vi "Named_Serial_Comms.vi"(0 "Channel Name":string, 1 "Write":string, 2 "Timeout/ms":u32=500, 4 "!Error retries":i32=10, 6 "!Timeout retries":i32=3, 9 "Port Name":string, 11 "Term Grep":string="\r$", 12 "Log Errors?":bool=TRUE, 13 "Terminate Count":i32) -> (3 "Read":string="This is simulation mode", 10 "millisecond timer value":u32, 14 "Timed out":bool, 15 "Serial Error":bool)   [LabVIEW 2016]
doc: "The Serial Communication VI performs bidirectional communication with a port. It initializes the port, writes a string to the port, and performs a read with timeout. The Read with Timeout will wait until a terminating character is received or the time limit is up, whichever comes first.\nThe initialisation parameters, terminating character, and timeout, are all set in the Serial Setup Global."
uses:
  Port_Params.ctl
  <vilib>/Instr/_visa.llb/VISA Find Search Mode.ctl
  <vilib>/Instr/serial.llb/serpConfig.vi
panel:
  in  "Tab Control":T1(tab)
  in  "Uppercase?":bool
  in  "Append Return?":bool
  in  "!stop":bool
  out "Terminated?":bool
  in  "Force setup reload":bool
  in  "Save Setups?":bool
  out "Buffer Trash":string
  out "byte count":u32
  out "Error Description":string
  out "Port Settings Array":T2[](array[typedef]) {"flow control etc."."parity err byte" format="%.0x"; "flow control etc."."XON byte" format="%.0x"; "flow control etc."."XOFF byte" format="%.0x"; "data bits" min=5 max=8 step=1}
  out "enumerated ports":string[](array[string])
  out "Ports having file settings":string[](array[string])
  out "Port Initialised?":bool[](array[boolean])
  out "Setting Number":i32
  out "Port Initialisation Parameters":T2={"Name"="", "flow control etc."={"input XON/XOFF"=FALSE, "input HW Handshake"=FALSE, "input alt HW HShk"=FALSE, "output XON/XOFF"=FALSE, "output HW Handshake"=FALSE, "output alt HW HShk"=FALSE, "XOFF byte "=0, "XON byte"=0, "parity err byte"=0}, "buffer size"=0, "baud rate"=9600, "data bits"=8, "stop bits"=enum."1 bit", "parity"=enum."no parity"} {"flow control etc."."parity err byte" format="%.0x"; "flow control etc."."XON byte" format="%.0x"; "flow control etc."."XOFF byte" format="%.0x"; "data bits" min=5 max=8 step=1}
  out "isGillUsonic":bool
  out "etherComms":errorcluster
  out "Audit trail":string[](array[string])
  out "Case":string="Simulate"
  out "Initialise error":i32
  out "Write error":i32
  out "n-bytes error code":i32
  out "read error code":i32
  out "Close Port error":i32
  out "load setups error":bool
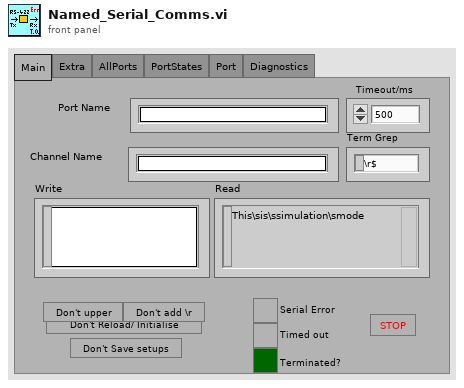
[diagram p1: front panel]
types:
  T1 = enum32{"Main", "Extra", "AllPorts", "PortStates", "Port", "Diagnostics"}
  T2 = typedef "Port_Params.ctl" = cluster{"Name":string, "flow control etc.":cluster{"input XON/XOFF":bool, "input HW Handshake":bool, "input alt HW HShk":bool, "output XON/XOFF":bool, "output HW Handshake":bool, "output alt HW HShk":bool, "XOFF byte ":u8, "XON byte":u8, "parity err byte":u16}, "buffer size":u16, "baud rate":u32, "data bits":u16, "stop bits":enum16{"1 bit", "1.5 bits", "2 bits"}, "parity":enum16{"no parity", "odd parity", "even parity", "mark parity", "space parity"}}
  T3 = enum16{"Standard", "Buffered", "CRLF", "Immediate"}
  T4 = typedef "VISA Find Search Mode.ctl" = u32
  T5 = cluster{"input XON/XOFF":bool, "input HW Handshake":bool, "input alt HW HShk":bool, "output XON/XOFF":bool, "output HW Handshake":bool, "output alt HW HShk":bool, "XOFF byte ":u8, "XON byte":u8, "parity err byte":u16}
  T6 = enum16{"no parity", "odd parity", "even parity", "mark parity", "space parity"}
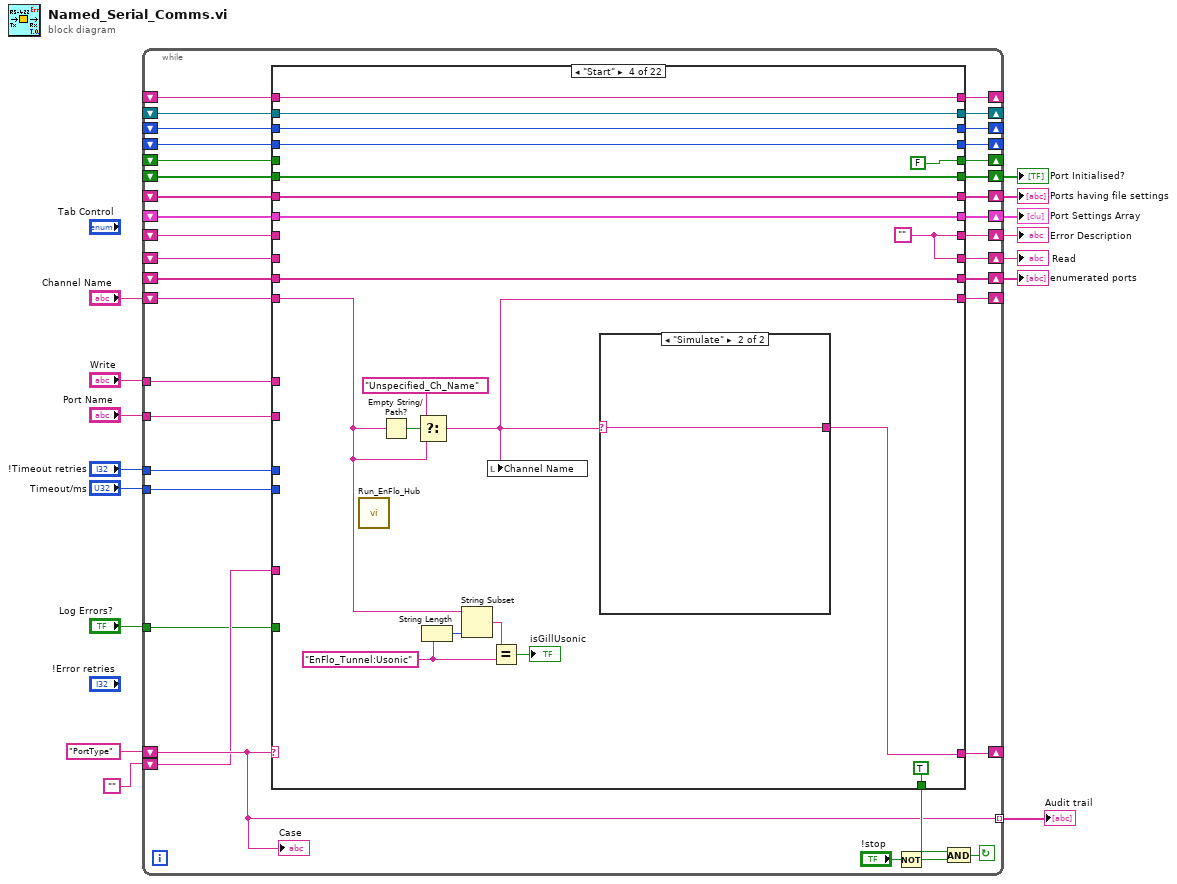
[diagram p0: block diagram]
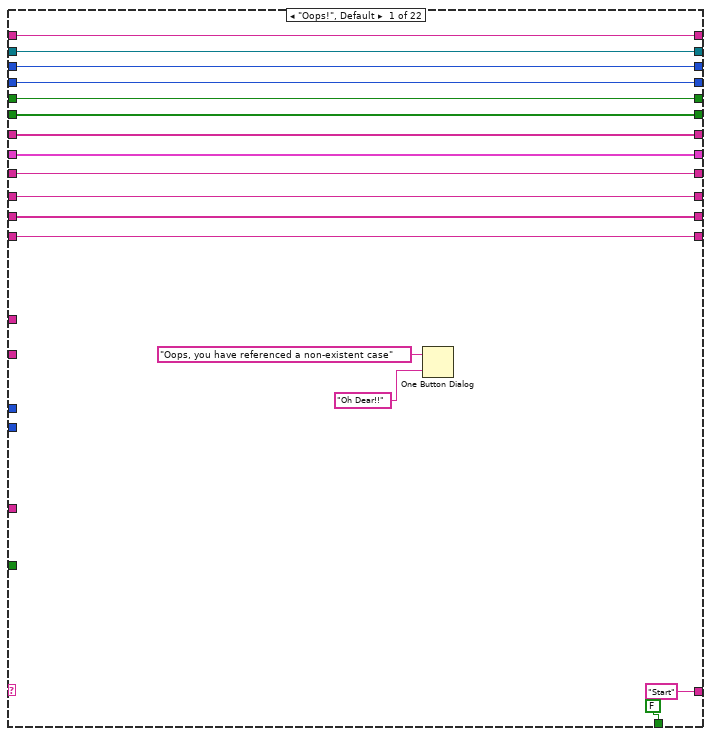
[diagram p2: hidden frame]
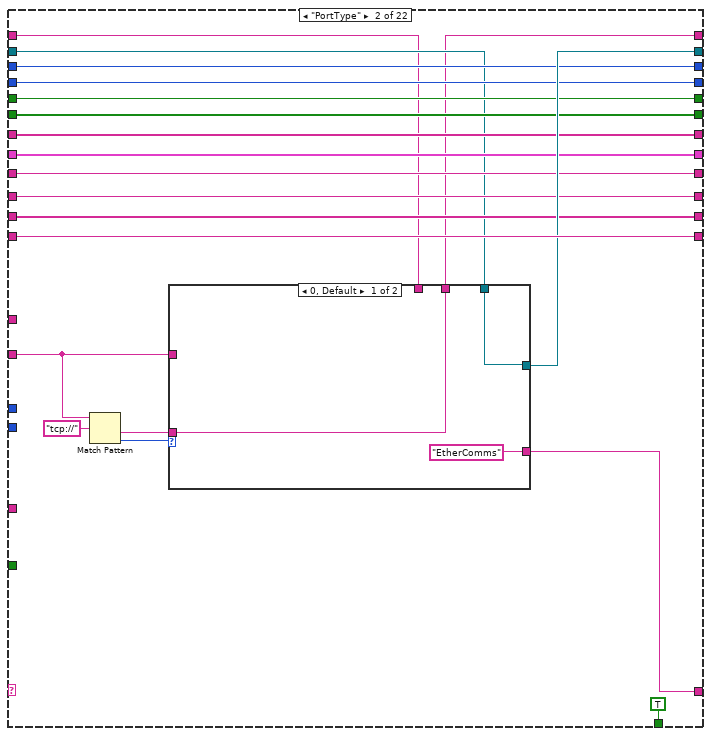
[diagram p3: hidden frame]
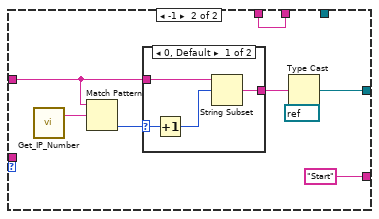
[diagram p4: hidden frame]
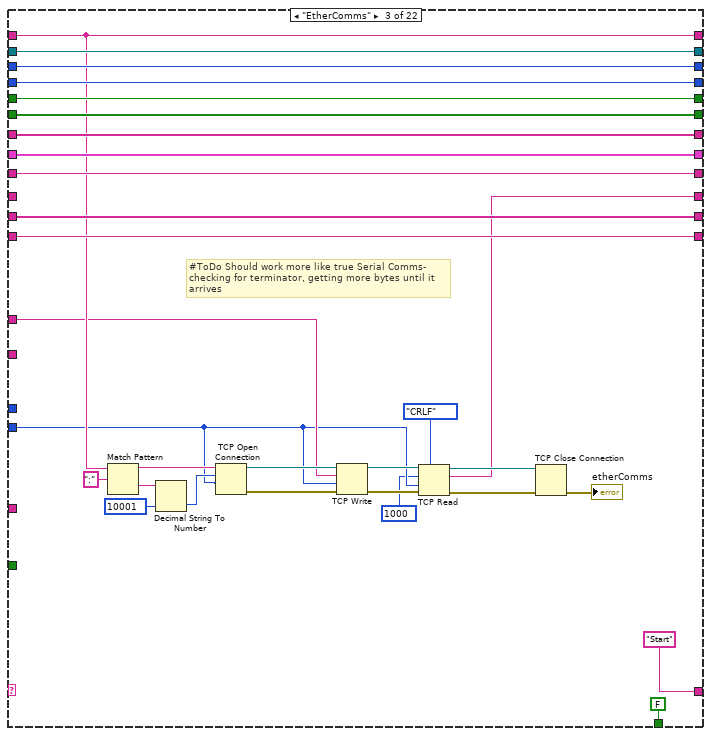
[diagram p6: hidden frame]
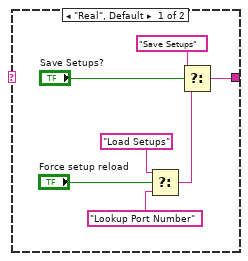
[diagram p7: hidden frame]
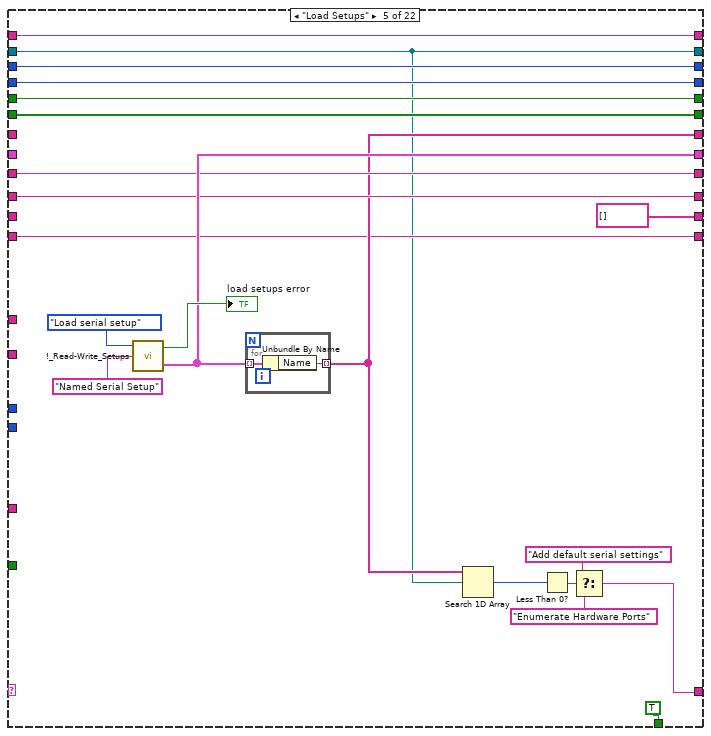
[diagram p8: hidden frame]
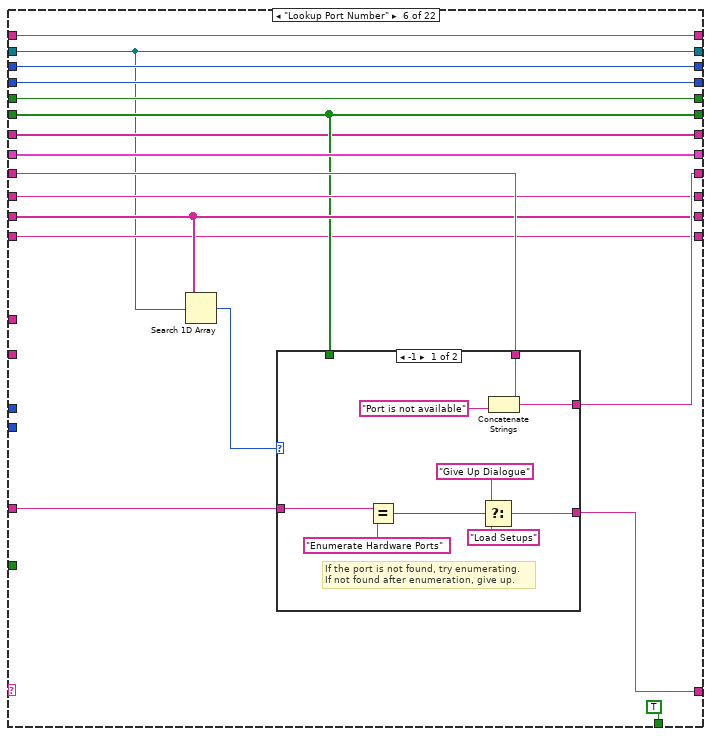
[diagram p9: hidden frame]
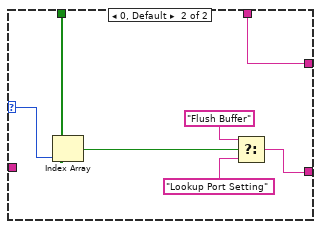
[diagram p10: hidden frame]
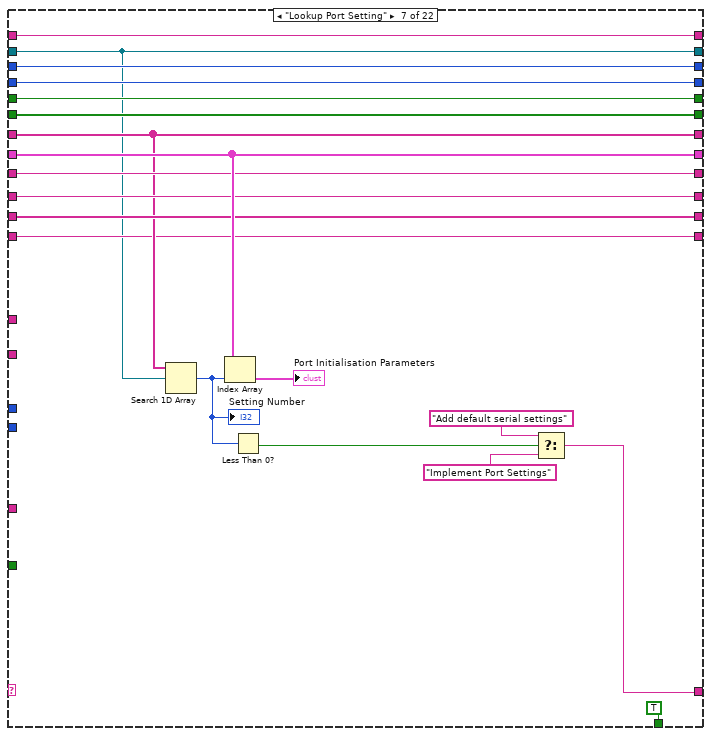
[diagram p11: hidden frame]
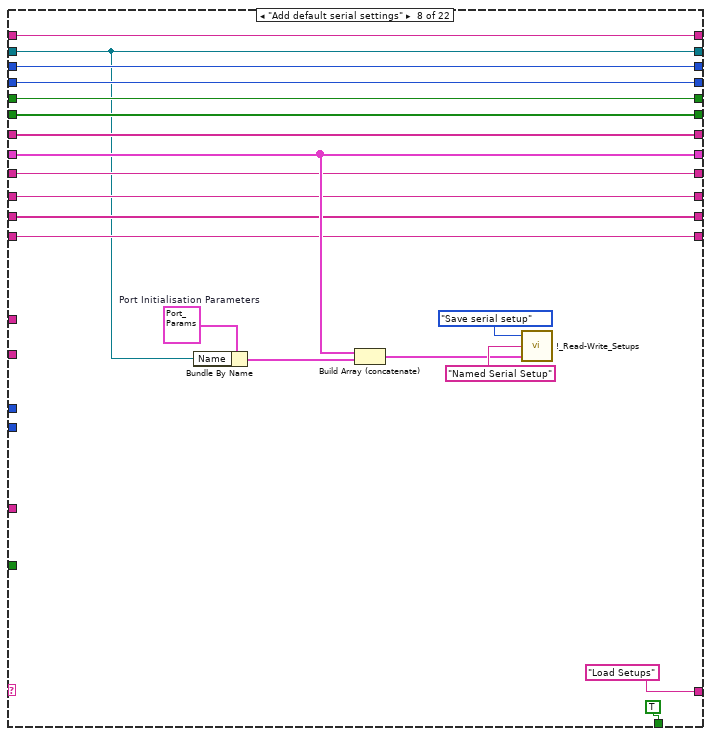
[diagram p12: hidden frame]
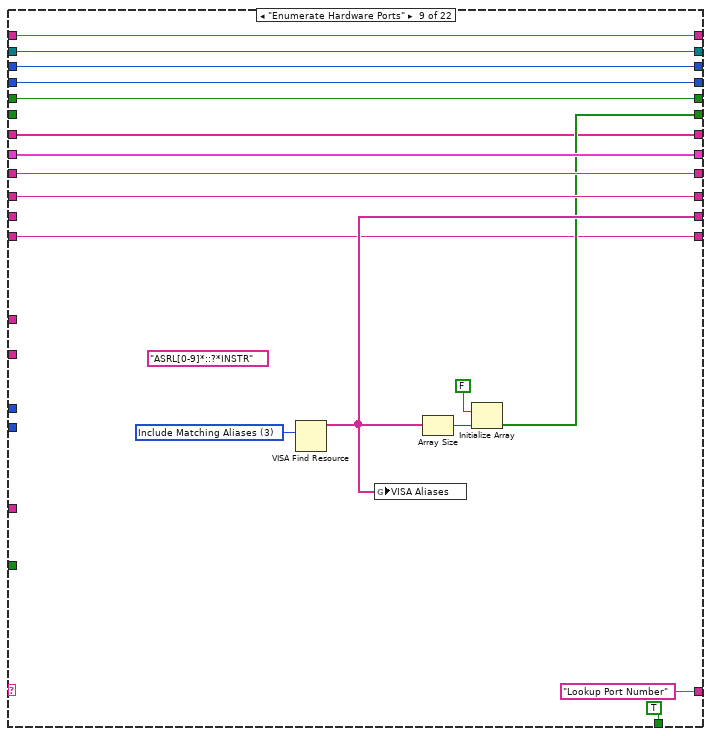
[diagram p13: hidden frame]
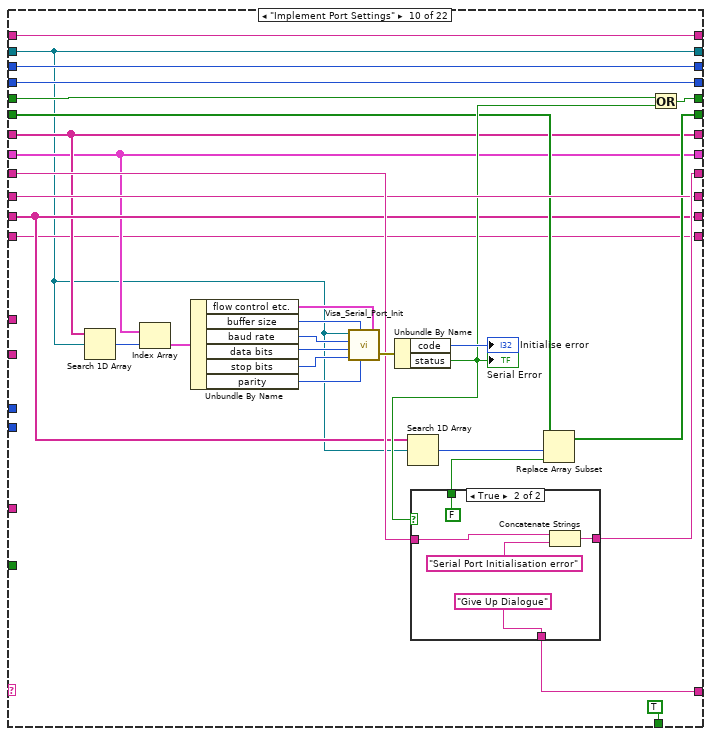
[diagram p14: hidden frame]
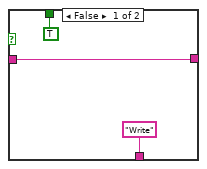
[diagram p15: hidden frame]
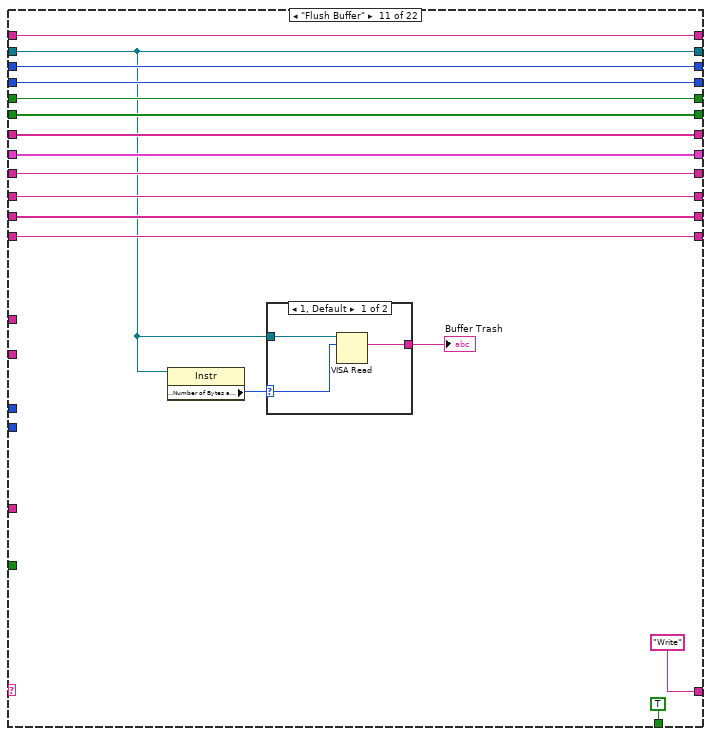
[diagram p16: hidden frame]
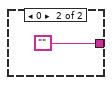
[diagram p17: hidden frame]
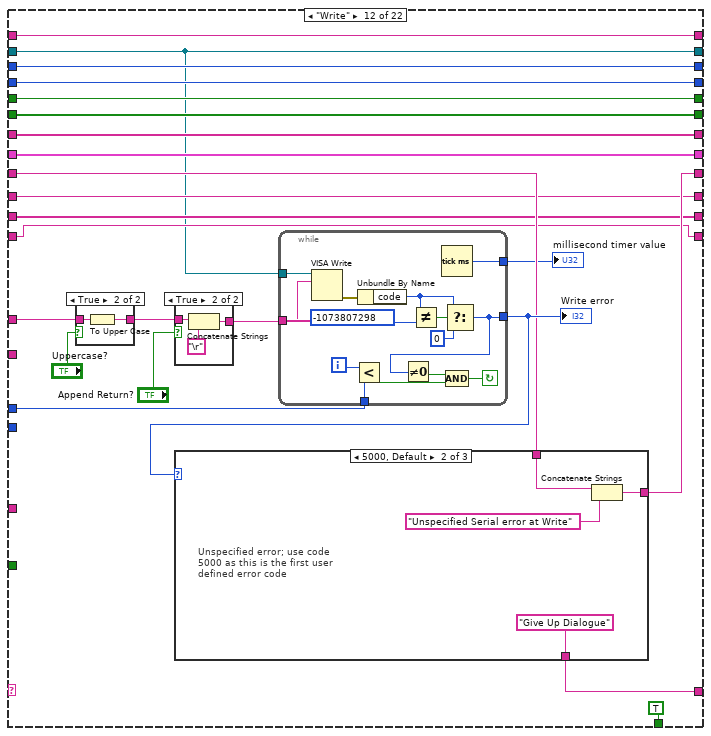
[diagram p18: hidden frame]
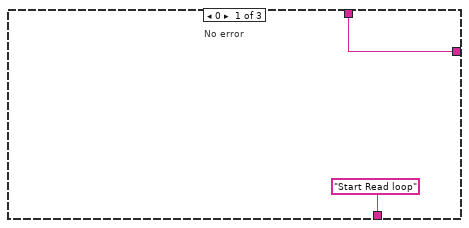
[diagram p19: hidden frame]
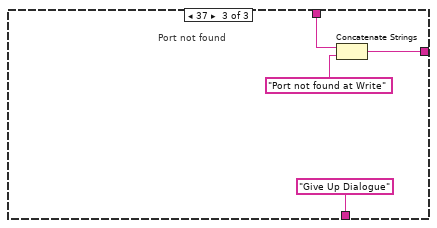
[diagram p20: hidden frame]
diagram:
  n1 = while {
    tunnel: "!Timeout retries" -> [w43]
    shift-left: "" -> [w44]
    tunnel: [w45] -> w3 mode=indexing
    shift-left: "PortType" -> [w45]
    shift-right: [w46] -> _
    tunnel: "Write" -> [w51]
    tunnel: "Log Errors?" -> [w42]
    shift-right: [w41] -> w10
    shift-left: _ -> [w40]
    shift-right: [w38] -> w9
    shift-left: _ -> [w39]
    shift-right: [w37] -> w8
    shift-left: _ -> [w36]
    shift-right: [w35] -> w7
    shift-left: _ -> [w34]
    shift-right: [w33] -> _
    shift-left: _ -> [w32]
    shift-right: [w31] -> w6
    shift-left: _ -> [w30]
    shift-right: [w28] -> w5
    shift-left: _ -> [w29]
    shift-right: [w25] -> _
    shift-left: _ -> [w24]
    shift-right: [w27] -> _
    shift-left: _ -> [w26]
    shift-right: [w22] -> _
    shift-left: "Channel Name" -> [w23]
    shift-right: [w21] -> _
    shift-left: _ -> [w20]
    tunnel: "Port Name" -> [w19]
    shift-right: [w18] -> _
    shift-left: _ -> [w17]
    tunnel: "Timeout/ms" -> [w16]
    stop <- w49 continue-if-true
    n2 = case shown="\"Start\"" w45 {
      tunnel: w51 -> [_ _ w109 _ _ _ _ _ _ _ _ w350 _ _ _ _ _ w532 w558 _ _ _]
      tunnel: ["Start" ("f") w68 "Start" w153 w164 w200 w220 "Load Setups" ("f") "Lookup Port Number" w295 "Write" ("f") w347 "Bytes At Serial Port?" ("f") w412 w454 w480 w522 "Start" "Start" "Start" "Start" ("f") "Load Setups" ("f")] -> w46
      tunnel: [FALSE TRUE FALSE TRUE TRUE TRUE TRUE TRUE TRUE TRUE TRUE TRUE TRUE TRUE TRUE TRUE TRUE FALSE FALSE TRUE FALSE TRUE] -> w50
      tunnel: w44 -> [_ _ _ _ _ w199 _ _ _ _ _ _ _ _ _ _ _ _ _ _ _ _]
      tunnel: w43 -> [_ _ _ _ _ _ _ _ _ _ _ w345 _ w411 _ _ _ _ _ _ _ _]
      tunnel: w42 -> [_ _ _ _ _ _ _ _ _ _ _ _ _ _ _ _ _ w538 _ _ _ _]
      tunnel: [w63 w80 w127 w151 w178 w198 w233 w248 w268 w279 w324 w344 w396 w410 w446 w473 w518 w537 w555 w574 w591 w605] -> w41
      tunnel: w40 -> [w63 w80 w127 w151 _ w198 w233 w248 w268 w279 w324 w344 w396 w410 w446 w473 w518 w537 w555 w574 w591 w605]
      tunnel: w39 -> [w62 w79 w126 _ w177 w197 w232 w247 w267 w290 w323 w342 w395 w409 w445 w472 w517 w536 w554 w573 w590 w604]
      tunnel: [w62 w79 w126 w150 w177 w196 w232 w247 w267 w291 w323 w343 w395 w409 w445 w472 w517 w536 w554 w573 w590 w604] -> w38
      tunnel: [w61 w78 w105 w150 w176 w195 w231 w246 w266 w289 w322 w341 "" w408 w444 w471 w516 w535 w553 w572 "Simulated Serial Read" w603] -> w37
      tunnel: w36 -> [w61 w78 _ _ w176 w195 w231 w246 w266 w289 w322 w341 _ w408 w443 w471 w516 w535 w553 w572 _ w603]
      tunnel: [w60 w77 w125 w149 string[] [] ("enumerated ports") w194 w230 w245 w265 w281 w321 w340 w393 w407 w442 w470 w515 w534 w552 w571 w588 w602] -> w35
      tunnel: w34 -> [w60 w77 w125 w149 _ w194 w230 w245 _ w281 w321 w340 w393 w407 w442 w470 w515 w534 w552 w571 w588 w602]
      tunnel: [w59 w83 w130 FALSE w174 w193 w229 w244 w264 w287 w318 w339 w392 w406 w441 w469 w513 w533 w551 w570 w587 w601] -> w33
      tunnel: w32 -> [w59 w83 w130 _ w174 w193 w229 w244 w264 w288 w318 w339 w392 w406 w441 w469 w514 w533 w551 w570 w587 w601]
      tunnel: [w58 w82 w129 w147 w173 w191 w228 w243 w263 w284 w317 w338 w391 w405 w440 w468 w511 w531 w550 w569 w586 w600] -> w31
      tunnel: w30 -> [w58 w82 w129 w147 w173 w191 w228 w243 _ w283 w317 w338 w391 w405 w440 w468 w511 w531 w550 w569 w586 w600]
      tunnel: [w57 w81 w128 w146 w172 w190 w227 w242 w262 w280 w316 w337 w390 w404 w439 w467 w510 w530 w549 w568 w585 w599] -> w28
      tunnel: w29 -> [w57 w81 w128 w146 _ w190 w227 w242 w262 w280 w316 w337 w390 w404 w439 w467 w510 w530 w549 w568 w585 w599]
      tunnel: [w56 w85 w132 w145 w171 w189 w226 w241 w261 w277 w315 w336 w389 w402 w435 w466 w509 w529 w548 w567 w584 w598] -> w27
      tunnel: w26 -> [w56 w85 w132 w145 w171 w189 w226 w241 w261 w277 w315 w336 _ w402 w435 w466 w509 w529 w548 w567 w584 w598]
      tunnel: [w55 w84 w131 w144 w170 w188 w225 w240 w260 w276 w314 w335 w388 w403 w434 w465 w508 w528 w547 w566 w583 w597] -> w25
      tunnel: w24 -> [w55 w84 w131 w144 w170 w188 w225 w240 w260 w276 w314 w335 w388 _ w434 w465 w508 w528 w547 w566 w583 w597]
      tunnel: w23 -> [w54 w87 w133 w136 w169 w187 w224 w239 w258 w275 w313 w333 w387 w401 w433 w464 w507 w527 w543 w565 w582 w596]
      tunnel: [w54 w87 w133 w134 w169 w187 w224 w239 w258 w275 w313 w333 w387 w401 w433 w464 w507 w527 w543 w565 w582 w596] -> w22
      tunnel: [w53 w86 w122 w141 w163 w186 w219 w238 w257 w274 w312 w332 w386 w400 w432 w463 w506 w526 w542 w564 w581 w595] -> w21
      tunnel: w20 -> [w53 w71 w122 w141 w163 w186 w219 w238 w257 w274 w312 w332 w386 w400 w432 w463 w506 w526 w542 w564 w581 w595]
      tunnel: w19 -> [_ w75 _ _ _ _ _ _ _ _ _ _ _ _ _ _ _ _ _ _ _ _]
      tunnel: [w52 w70 w115 w140 w162 w185 w218 w237 w256 w273 w311 w331 w385 w399 w431 w462 w505 w525 w541 w563 w580 w594] -> w18
      tunnel: w17 -> [w52 w69 w115 w140 w162 w185 w218 w237 w256 w273 w311 w331 w385 w399 w431 w462 w505 w525 w541 w563 w580 w594]
      tunnel: w16 -> [_ _ w108 _ _ _ _ _ _ _ _ _ _ _ _ _ w504 _ _ _ _ _]
      frame "Oops!", Default {
        n3 = One Button Dialog(message="Oops, you have referenced a non-existent case", button name ("OK")="Oh Dear!!") -> ()  [unwired: 1 out]
      }
      frame "PortType" {
        n4 = Match Pattern(string=w75, regular expression="tcp://") -> (after substring=w72:string, offset past match=w73:i32)  [unwired: 1 in, 2 out]
        n5 = case shown="0, Default" w73 {
          tunnel: [w90 w94] -> w86
          tunnel: w75 -> [_ w93]
          tunnel: w72 -> [w89 _]
          tunnel: w71 -> [w90 _]
          tunnel: [w89 w92] -> w70
          tunnel: w69 -> [_ w92]
          tunnel: ["EtherComms" "Start"] -> w68
          frame 0, Default {
          }
          frame -1 {
            n6 = call "Get_IP_Number.vi"() -> ("IP Number"=w97:string)  [unwired: 1 out]
            n7 = Match Pattern(string=w93, regular expression=w97) -> (offset past match=w96:i32)  [unwired: 4 out]
            n8 = case shown="0, Default" w96 {
              selector: w96 -> [w99 _]
              tunnel: [w100 w103] -> w98
              tunnel: w93 -> [w101 w103]
              frame 0, Default {
                n9 = Increment(x=w99) -> (x+1=w102:i32)
                n10 = String Subset(string=w101, offset (0)=w102) -> (substring=w100:string)  [unwired: 1 out]
              }
              frame -1 {
              }
            }
            n11 = Type Cast(type=refnum<visa-resource-name> refnum ("dup VISA resource name"), x=w98) -> (*(type *) &x=w94:refnum<visa-resource-name>)
          }
        }
      }
      frame "EtherComms" {
        # "#ToDo Should work more like true Serial Comms- checking for terminator, getting more bytes until it arrives"
        n12 = Match Pattern(string=w115, regular expression=":") -> (before substring=w113:string, after substring=w112:string)  [unwired: 1 in, 2 out]
        n13 = Decimal String To Number(string=w112, default (0L)=u16 10001 ("default (0 I32)")) -> (number=w111:u16)  [unwired: 1 in, 1 out]
        n14 = TCP Open Connection(address=w113, remote port or service name=w111, timeout ms (60000)=w108) -> (connection ID=w116:refnum<k5>, error out=w119:errorcluster)  [unwired: 2 in]
        n15 = TCP Write(connection ID=w116, data in=w109, error in (no error)=w119, 9:w108) -> (connection ID out=w117:refnum<k5>, error out=w118:errorcluster)  [unwired: 1 out]
        n16 = TCP Read(connection ID=w117, bytes to read=1000, error in (no error)=w118, 7:T3."CRLF" ("mode (standard)"), 9:w108) -> (connection ID out=w121:refnum<k5>, data out=w105:string, error out=w120:errorcluster)
        n17 = TCP Close Connection(connection ID=w121, error in (no error)=w120) -> (error out=→"etherComms":errorcluster)  [unwired: 1 in, 1 out]
      }
      frame "Start" {
        w139 = "EnFlo_Tunnel:Usonic"
        w150 = ""
        n18 = call "Run_EnFlo_Hub.vi"() -> ()  [unwired: 1 in, 7 out]
        n19 = Empty String/Path?(string/path=w136) -> (empty?=w143:bool)
        n20 = Select(t="Unspecified_Ch_Name", s=w143, f=w136) -> (s? t:f=w134:string)
        n21 = String Length(string=w139) -> (length=w137:i32)
        n22 = String Subset(string=w136, length (rest)=w137) -> (substring=w138:string)  [unwired: 1 out]
        n23 = local write "Channel Name"(w134) -> ()
        n24 = Equal?(x=w138, y=w139) -> (x = y?=→"isGillUsonic":bool)
        n25 = case shown="\"Simulate\"" w134 {
          selector: w134 -> [_ w161]
          tunnel: [w156 w161] -> w153
          frame "Real", Default {
            n26 = Select(t="Load Setups" ("f"), s="Force setup reload", f="Lookup Port Number") -> (s? t:f=w157:string)
            n27 = Select(t="Save Setups", s="Save Setups?", f=w157) -> (s? t:f=w156:string)
          }
          frame "Simulate" {
          }
        }
      }
      frame "Load Setups" {
        n28 = call "!_Read-Write_Setups.vi"("Setup Name"="Named Serial Setup", "Mode"=enum16{"Load serial setup", "Save serial setup"}."Load serial setup") -> ("Port Settings Array Out"=w178:T2[], "error unflattening"=→"load setups error":bool)  [unwired: 1 in]
        n29 = for {
          tunnel: w178 -> [w184] mode=indexing
          tunnel: [w183] -> w172 mode=indexing
          n30 = Unbundle By Name(w184) -> ("Name"=w183:string)
        }
        n31 = Search 1D Array(1D array=w172, element=w163) -> (index of element=w168:i32)  [unwired: 1 out]
        n32 = Less Than 0?(x=w168) -> (x < 0?=w167:bool)
        n33 = Select(t="Add default serial settings", s=w167, f="Enumerate Hardware Ports") -> (s? t:f=w164:string)
      }
      frame "Lookup Port Number" {
        n34 = Search 1D Array(1D array=w194, element=w186) -> (index of element=w192:i32)  [unwired: 1 out]
        n35 = case shown="-1" w192 {
          selector: w192 -> [_ w211]
          tunnel: [w210 w217] -> w200
          tunnel: w199 -> [w207 _]
          tunnel: w197 -> [w203 w213]
          tunnel: [w202 w213] -> w196
          tunnel: w191 -> [_ w212]
          frame -1 {
            # "If the port is not found, try enumerating.\nIf not found after enumeration, give up."
            n36 = Equal?(x=w207, y="Enumerate Hardware Ports" ("f")) -> (x = y?=w209:bool)
            n37 = Select(t="Give Up Dialogue" ("f"), s=w209, f="Load Setups") -> (s? t:f=w210:string)
            n38 = Concatenate Strings(w203, "Port is not available" ("Error Description")) -> (w202:string)
          }
          frame 0, Default {
            n39 = Index Array(array=w212, index=w211) -> (element=w216:bool)
            n40 = Select(t="Flush Buffer" ("f"), s=w216, f="Lookup Port Setting") -> (s? t:f=w217:string)
          }
        }
      }
      frame "Lookup Port Setting" {
        n41 = Search 1D Array(1D array=w227, element=w219) -> (index of element=w234:i32)  [unwired: 1 out]
        "Setting Number" <- w234
        n42 = Index Array(array=w233, index=w234) -> (element=→"Port Initialisation Parameters":T2)
        n43 = Less Than 0?(x=w234) -> (x < 0?=w223:bool)
        n44 = Select(t="Add default serial settings", s=w223, f="Implement Port Settings") -> (s? t:f=w220:string)
      }
      frame "Add default serial settings" {
        w255 = T2 {"Name"="", "flow control etc."={"input XON/XOFF"=FALSE, "input HW Handshake"=FALSE, "input alt HW HShk"=FALSE, "output XON/XOFF"=FALSE, "output HW Handshake"=FALSE, "output alt HW HShk"=FALSE, "XOFF byte "=19, "XON byte"=17, "parity err byte"=0}, "buffer size"=200, "baud rate"=9600, "data bits"=8, "stop bits"=enum."1 bit", "parity"=enum."no parity"}  # Port Initialisation Parameters
        n45 = Bundle By Name(cluster=w255, "Name"=w238) -> (w254:T2)
        n46 = Build Array (concatenate)(w248, w254) -> (w251:T2[])
        n47 = call "!_Read-Write_Setups.vi"("Port Settings Array In"=w251, "Setup Name"="Named Serial Setup", "Mode"=enum16{"Load serial setup", "Save serial setup"}."Save serial setup") -> ()  [unwired: 2 out]
      }
      frame "Enumerate Hardware Ports" {
        w259 = T4 3 items=["Canonical Names Only"=0, "Aliases Only"=2, "Include Matching Aliases"=3, "Include All Aliases"=4] ("Search Mode")
        (unwired) "ASRL[0-9]*::?*INSTR" ("expression (\"?*\")")
        n48 = VISA Find Resource(10:w259) -> (3:w265:string[])  [unwired: 1 in, 3 out]
        n49 = global write "serpConfig.vi" "VISA Aliases"(w265) -> ()
        n50 = Array Size(array=w265) -> (size(s)=w270:i32)
        n51 = Initialize Array(FALSE, w270) -> (w263:bool[])
      }
      frame "Implement Port Settings" {
        n52 = Search 1D Array(1D array=w280, element=w274) -> (index of element=w282:i32)  [unwired: 1 out]
        n53 = Index Array(array=w279, index=w282) -> (element=w278:T2)
        n54 = Unbundle By Name(w278) -> ("flow control etc."=w302:T5, "buffer size"=w301:u16, "baud rate"=w300:u32, "data bits"=w299:u16, "stop bits"=w298:enum16{"1 bit", "1.5 bits", "2 bits"}, "parity"=w297:T6)
        n55 = call "Visa_Serial_Port_Init.vi"("flow control etc."=w302, "parity"=w297, "buffer size"=w301, "stop bits"=w298, "data bits"=w299, "baud rate"=w300, "Visa Port Name"=w274) -> ("error out"=w293:errorcluster)
        n56 = Unbundle By Name(w293) -> ("code"=→"Initialise error":i32, "status"=w286:bool)
        "Serial Error" <- w286
        n57 = Search 1D Array(1D array=w281, element=w274) -> (index of element=w285:i32)  [unwired: 1 out]
        n58 = case shown="True" w286 {
          tunnel: ["Write" "Give Up Dialogue"] -> w295
          tunnel: [TRUE ("Element Data") FALSE ("Element Data")] -> w294
          tunnel: [w303 w307] -> w291
          tunnel: w290 -> [w303 w306]
          frame False {
          }
          frame True {
            n59 = Concatenate Strings(w306, "Serial Port Initialisation error" ("Error Description")) -> (w307:string)
          }
        }
        n60 = Replace Array Subset(array=w283, new element=w294, index=w285) -> (w284:bool[])
        n61 = Or(x=w288, y=w286) -> (x .or. y?=w287:bool)
      }
      frame "Flush Buffer" {
        n62 = property class="Instr"(reference=w312) -> ("Serial Settings:Number of Bytes at Serial Port"=w320:u32)  [unwired: 1 in, 2 out]
        n63 = case shown="1, Default" w320 {
          selector: w320 -> [w327 _]
          tunnel: [w329 ""] -> w319
          tunnel: w312 -> [w328 _]
          frame 1, Default {
            n64 = VISA Read(VISA resource name=w328, byte count=w327) -> (read buffer=w329:string)  [unwired: 1 in, 3 out]
          }
          frame 0 {
          }
        }
        "Buffer Trash" <- w319
      }
      frame "Write" {
        n65 = case shown="True" "Uppercase?" {
          tunnel: w350 -> [w382 w384]
          tunnel: [w382 w383] -> w352
          frame False {
          }
          frame True {
            n66 = To Upper Case(1:w384) -> (0:w383:string)
          }
        }
        n67 = case shown="True" "Append Return?" {
          tunnel: w352 -> [w378 w381]
          tunnel: [w378 w380] -> w349
          frame False {
          }
          frame True {
            n68 = Concatenate Strings(w381, "\r") -> (w380:string)
          }
        }
        n69 = while {
          tunnel: w345 -> [w363]
          tunnel: [w354] -> w346
          tunnel: w349 -> [w361]
          tunnel: w332 -> [w360]
          tunnel: [w359] -> w334
          i -> [w367]
          stop <- w364 continue-if-true
          n70 = VISA Write(VISA resource name=w360, write buffer=w361) -> (error out=w362:errorcluster)  [unwired: 1 in, 2 out]
          n71 = Less?(x=w367, y=w363) -> (x < y?=w366:bool)
          n72 = Unbundle By Name(w362) -> ("code"=w356:i32)
          n73 = Not Equal?(x=w356, y=-1073807298 ("code")) -> (x != y?=w357:bool)
          n74 = Tick Count (ms)() -> (millisecond timer value=w359:u32)
          n75 = Select(t=w356, s=w357, f=0) -> (s? t:f=w354:i32)
          n76 = Not Equal To 0?(x=w354) -> (x != 0?=w365:bool)
          n77 = Compound Arithmetic op=AND(w365, w366) -> (w364:bool)
        }
        "Write error" <- w346
        "millisecond timer value" <- w334
        n78 = case shown="5000, Default" w346 {
          tunnel: ["Start Read loop" "Give Up Dialogue" "Give Up Dialogue"] -> w347
          tunnel: [w368 w371 w374] -> w343
          tunnel: w342 -> [w368 w370 w376]
          frame 0 {
            # "No error"
          }
          frame 5000, Default {
            # "Unspecified error; use code 5000 as this is the first user defined error code"
            n79 = Concatenate Strings(w370, "Unspecified Serial error at Write" ("Error Description")) -> (w371:string)
          }
          frame 37 {
            # "Port not found"
            n80 = Concatenate Strings(w376, "Port not found at Write" ("Error Description")) -> (w374:string)
          }
        }
      }
      frame "Start Read loop" {
        n81 = Tick Count (ms)() -> (millisecond timer value=w389:u32)
      }
      frame "Bytes At Serial Port?" {
        # "#Yuk Shouldn't use \"Timeout retries\" to say how many times to check for bytes at port!"
        n82 = while {
          tunnel: w411 -> [w421]
          tunnel: [w418] -> w403
          tunnel: [w422] -> w415
          tunnel: w400 -> [w419]
          i -> [w425]
          stop <- w423 continue-if-true
          n83 = property class="Instr"(reference=w419) -> (error out=w417:errorcluster, "Serial Settings:Number of Bytes at Serial Port"=w418:u32)  [unwired: 1 in, 1 out]
          "byte count" <- w418
          n84 = Unbundle By Name(w417) -> ("code"=w420:i32)
          "n-bytes error code" <- w420
          n85 = Less?(x=w425, y=w421) -> (x < y?=w424:bool)
          n86 = Equal To 0?(x=w420) -> (x = 0?=w422:bool)
          n87 = Compound Arithmetic op=AND(invert w422, w424) -> (w423:bool)
          n88 = case shown="True" w423 {
            frame False {
            }
            frame True {
              n89 = Wait (ms)(milliseconds to wait=u32 5) -> ()  [unwired: 1 out]
            }
          }
        }
        n90 = case shown="0" w403 {
          tunnel: ["Serial Port Read" ("f") "Check for Termination" ("f")] -> w413
          frame 1, Default {
          }
          frame 0 {
            n91 = Wait (ms)(milliseconds to wait=u32 1) -> ()  [unwired: 1 out]
          }
        }
        n92 = Select(t=w413, s=w415, f="Log") -> (s? t:f=w412:string)
      }
      frame "Serial Port Read" {
        n93 = local read "isGillUsonic"() -> (w430:bool)
        n94 = Greater?(x=w434, y=u32 1) -> (0:w450:bool)
        n95 = And(x=w450, y=w430) -> (x .and. y?=w449:bool)
        n96 = case shown="False" w449 {
          tunnel: w434 -> [w459 w461]
          tunnel: [w459 w460] -> w436
          frame False {
          }
          frame True {
            n97 = Decrement(x=w461) -> (x-1=w460:u32)
          }
        }
        n98 = VISA Read(VISA resource name=w432, byte count=w436) -> (read buffer=w437:string, error out=w438:errorcluster)  [unwired: 1 in, 2 out]
        n99 = Unbundle By Name(w438) -> ("code"=w448:i32)
        n100 = case shown="1073676294" w448 {
          selector: w448 -> [w457 _]
          tunnel: [w457 0 ("code")] -> w447
          frame 0, Default {
          }
          frame 1073676294 {
          }
        }
        "read error code" <- w447
        n101 = Concatenate Strings(w443, w437) -> (w444:string)
        n102 = Equal To 0?(x=w447) -> (x = 0?=w453:bool)
        n103 = Select(t="Check for Termination" ("f"), s=w453, f="Log") -> (s? t:f=w454:string)
      }
      frame "Check for Termination" {
        n104 = Empty String/Path?(string/path="Term Grep") -> (empty?=w482:bool)
        n105 = case shown="False" w482 {
          tunnel: "Terminate Count" -> [w486 w501]
          tunnel: w471 -> [w488 w502]
          tunnel: [w483 w500] -> w477
          tunnel: "Term Grep" -> [w489 _]
          frame False {
            n106 = Decrement(x=w486) -> (x-1=w485:i32)
            n107 = while {
              tunnel: [w490] -> w484
              tunnel: w485 -> [w493]
              shift-left: 0 -> [w497]
              shift-right: [w496] -> _
              tunnel: w488 -> [w498]
              tunnel: w489 -> [w499]
              i -> [w494]
              stop <- w491 continue-if-true
              n108 = Match Pattern(string=w498, regular expression=w499, offset (0)=w497) -> (match substring=w490:string, offset past match=w496:i32)  [unwired: 2 out]
              n109 = Less?(x=w494, y=w493) -> (x < y?=w492:bool)
              n110 = Greater Or Equal To 0?(x=w496) -> (x >= 0?=w495:bool)
              n111 = Compound Arithmetic op=AND(w495, w492) -> (w491:bool)
            }
            n112 = Empty String/Path?(string/path=w484) -> (empty?=w483:bool)
          }
          frame True {
            n113 = String Length(string=w502) -> (length=w503:i32)
            n114 = Less?(x=w503, y=w501) -> (x < y?=w500:bool)
          }
        }
        n115 = Not(x=w477) -> (.not. x?=w474:bool)
        "Terminated?" <- w474
        n116 = Select(t="Log" ("f"), s=w474, f="TimeOut?") -> (s? t:f=w480:string)
      }
      frame "TimeOut?" {
        n117 = Tick Count (ms)() -> (millisecond timer value=w523:u32)
        n118 = Subtract(x=w523, y=w509) -> (x-y=w524:u32)
        n119 = Greater?(x=w524, y=w504) -> (0:w512:bool)
        "Timed out" <- w512
        n120 = Select(t="Log" ("f"), s=w512, f="Bytes At Serial Port?") -> (s? t:f=w522:string)
        n121 = Or(x=w514, y=w512) -> (x .or. y?=w513:bool)
      }
      frame "Log" {
        n122 = call "!_Serial_log_builder.vi"("Port Name"=w526, "Comms Error"=w533, "Write String"=w532, "Log Errors?"=w538, "Read"=w535) -> ()  [unwired: 1 in, 3 out]
      }
      frame "Give Up Dialogue" {
        n123 = Format Into String(format string="%s%s%s%s%s%s\" ", initial string=w554, " whilst trying to write \n\"", w558, "\" to Channel \"", w543, "\" at Port \"" ("Input 5"), w542) -> (resulting string=w546:string)  [unwired: 1 in, 1 out]
        n124 = call "Server_Emails.vi"("Message"=w546, "Contact All clients?"=TRUE, "Subject"="Serial_Comms_Error") -> ()  [unwired: 2 in, 3 out]
      }
      frame "Close All Ports" {
        n125 = for {
          tunnel: w571 -> [w577] mode=indexing
          n126 = VISA Close(VISA resource name=w577) -> (error out=w579:errorcluster)  [unwired: 1 in]
          n127 = Unbundle By Name(w579) -> ("code"=→"Close Port error":i32)
        }
      }
      frame "Simulate" {
        (unwired) "This is simulation mode" ("Read")
      }
      frame "Save Setups" {
        n128 = call "!_Read-Write_Setups.vi"("Port Settings Array In"=w605, "Setup Name"="Named Serial Setup", "Mode"=enum16{"Load serial setup", "Save serial setup"}."Save serial setup") -> ()  [unwired: 2 out]
      }
    }
    n129 = Not(x="!stop") -> (.not. x?=w47:bool)
    n130 = And(x=w50, y=w47) -> (x .and. y?=w49:bool)
    "Case" <- w45
  }
  "Port Settings Array" <- w10
  "Error Description" <- w9
  "Read" <- w8
  "enumerated ports" <- w7
  "Port Initialised?" <- w6
  "Ports having file settings" <- w5
  "Audit trail" <- w3
